vi "VeriStand DSF.Transfer.Configuration.Channel Data Ref to Offset.vi"(8 "error in (no error)":errorcluster, 11 "Channel Data Reference":T1 format="%.0x") -> (0 "error out":errorcluster, 3 "channel offset":u64)   [LabVIEW 2017, in "Data Sharing Framework Engine.lvlib" / "VeriStand DSF.Transfer.Configuration.lvclass"]
uses:
  VeriStand DSF.Transfer.Configuration.lvclass
  <vilib>/NI Veristand/Custom Device API/Data Reference.ctl
  <vilib>/NI VeriStand/Custom Device API/Custom Device API.lvlib
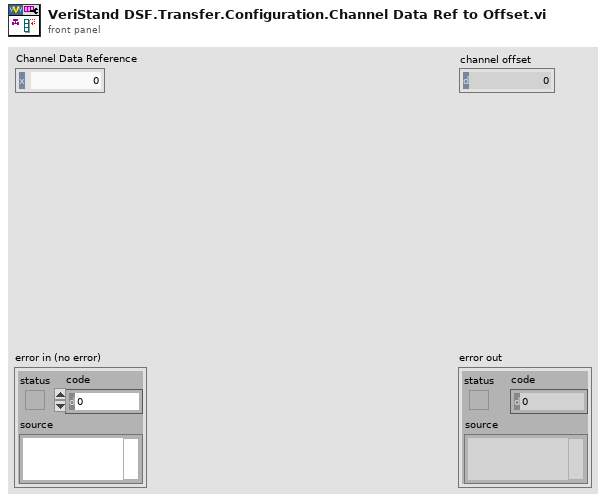
[diagram p1: front panel]
types:
  T1 = typedef "Custom Device API.lvlib/Data Reference.ctl" = i32
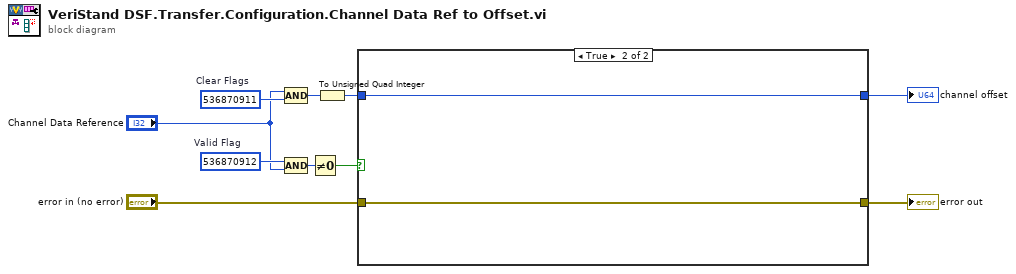
[diagram p0: block diagram]
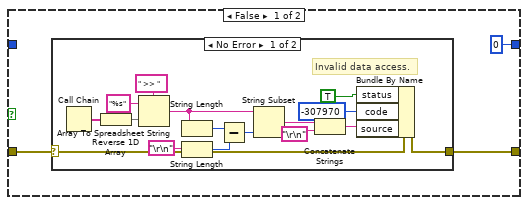
[diagram p2: hidden frame]
diagram:
  w8 = T1 536870912  # Valid Flag
  w9 = T1 536870911  # Clear Flags
  n1 = Compound Arithmetic op=AND("Channel Data Reference", w9) -> (w4:T1)
  n2 = Compound Arithmetic op=AND(w8, "Channel Data Reference") -> (w10:T1)
  n3 = Not Equal To 0?(x=w10) -> (x != 0?=w6:bool)
  n4 = To Unsigned Quad Integer(1:w4) -> (0:w3:u64)
  n5 = case shown="True" w6 {
    tunnel: w3 -> [_ w32]
    tunnel: "error in (no error)" -> [w12 w31]
    tunnel: [u64 0 w32] -> w2
    tunnel: [w11 w31] -> w1
    frame False {
      n6 = case shown="No Error" w12 {
        selector: w12 -> [w26 w30]
        tunnel: [w29 w30] -> w11
        frame No Error {
          # "Invalid data access."
          n7 = Call Chain() -> (call chain=w15:string[])
          n8 = Reverse 1D Array(array=w15) -> (reversed array=w22:string[])
          n9 = Array To Spreadsheet String(delimiter (Tab)=" >> ", array=w22, 3:"%s" ("format string")) -> (spreadsheet string=w23:string)
          n10 = String Length(string=w23) -> (length=w21:i32)
          n11 = String Length(string="\r\n") -> (length=w25:i32)
          n12 = Subtract(x=w21, y=w25) -> (x-y=w20:i32)
          n13 = String Subset(string=w23, length (rest)=w20) -> (substring=w16:string)  [unwired: 1 out]
          n14 = Concatenate Strings(w16, "\r\n") -> (w14:string)
          n15 = Bundle By Name(cluster=w26, "status"=TRUE, "code"=-307970, "source"=w14) -> (w29:errorcluster)
        }
        frame Error {
          # "Leave existing error."
        }
      }
    }
    frame True {
    }
  }
  "error out" <- w1
  "channel offset" <- w2
